vi "ReadPin.vi"(8 "error in (no error)":errorcluster, 9 "Pin":dbl, 10 "Port":dbl, 11 "Cypress in":refnum<class "Cypress.lvclass">) -> (0 "error out":errorcluster, 3 "Cypress out":refnum<class "Cypress.lvclass">)   [LabVIEW 2020, in "Cypress.lvclass"]
uses:
  Cypress.lvclass
  Cypress.lvclass/Cypress.ctl
  9febd328-30e5-4dc8-9827-3de5b44f5e7d.vi
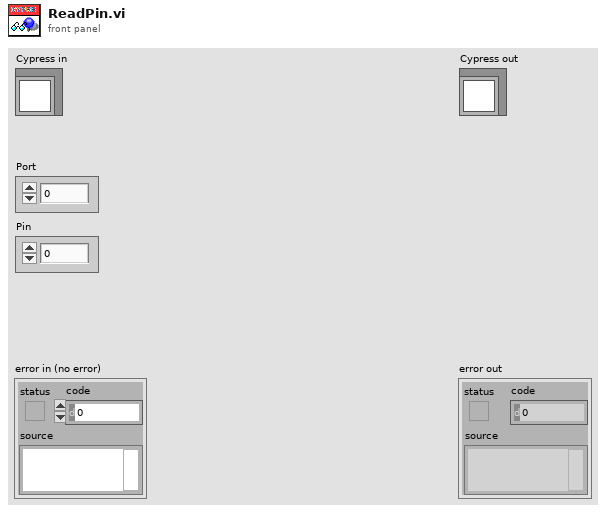
[diagram p1: front panel]
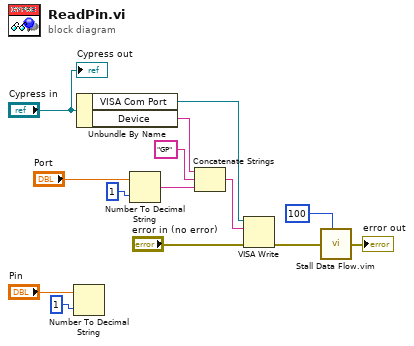
[diagram p0: block diagram]
diagram:
  n1 = Number To Decimal String(number="Pin", width (-)=i16 1) -> ()  [unwired: 1 out]
  n2 = Unbundle By Name("Cypress in") -> ("VISA Com Port"=w7:refnum<visa-resource-name>, "Device"=w6:string)
  n3 = Number To Decimal String(number="Port", width (-)=i16 1) -> (decimal integer string=w12:string)
  n4 = Concatenate Strings(w6, "GP" ("string"), w12) -> (w13:string)
  n5 = VISA Write(VISA resource name=w7, write buffer=w13, error in (no error)="error in (no error)") -> (error out=w14:errorcluster)  [unwired: 2 out]
  n6 = call "Stall Data Flow.vim"("value in"=w14, "milliseconds to wait"=u32 100) -> ("value out"=→"error out":errorcluster)  [unwired: 1 out]
  "Cypress out" <- "Cypress in"
